vi "Nested Loops Solution.vi"() -> (3 "Solutions (Quantity)":i32[][](array[numeric]))   [LabVIEW 2014]
uses:
  ctl/Coin data--cluster.ctl
panel:
  in  "Update display?":bool
  out "No. solutions":i32
  out "Values (p)":i32[](array[numeric])
  out "Progress - current iteration values":i32[](array[numeric])
  out "Time taken (s)":dbl
  # "Beer money - Nested Loops/ Speedy solution"
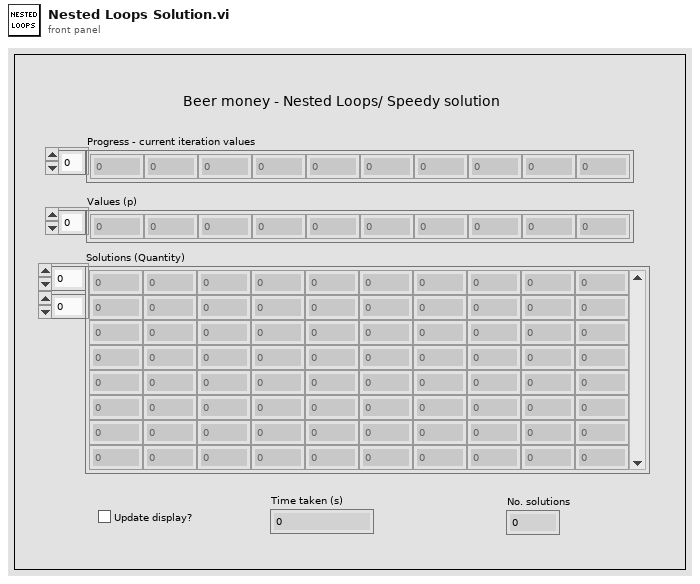
[diagram p1: front panel]
types:
  T1 = typedef "Coin data--cluster.ctl" = cluster{"Coin/note":i32, "Quantity":i32}
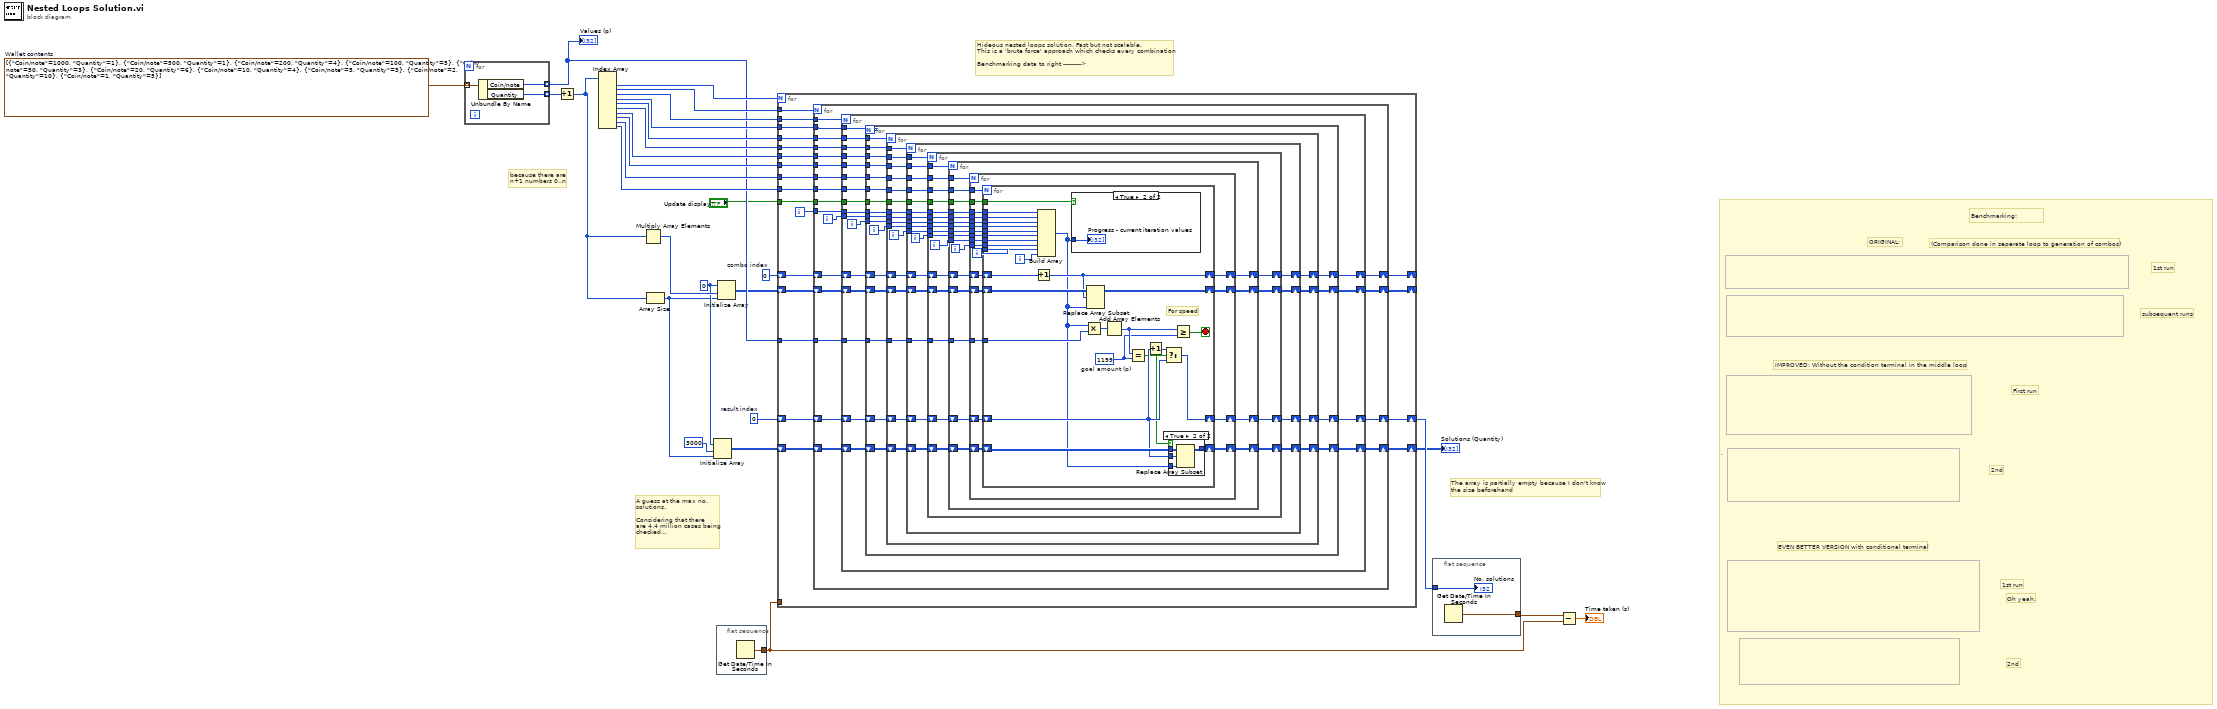
[diagram p0: block diagram]
diagram:
  w5 = 0 ("dimension size")
  w9 = 0  # result index
  w14 = 0  # combo index
  w28 = T1[] [{"Coin/note"=1000, "Quantity"=1}, {"Coin/note"=500, "Quantity"=1}, {"Coin/note"=200, "Quantity"=4}, {"Coin/note"=100, "Quantity"=5}, {"Coin/note"=50, "Quantity"=3}, {"Coin/note"=20, "Quantity"=6}, {"Coin/note"=10, "Quantity"=4}, {"Coin/note"=5, "Quantity"=3}, {"Coin/note"=2, "Quantity"=10}, {"Coin/note"=1, "Quantity"=5}]  # Wallet contents
  # "2nd"
  # "subsequent runs"
  # "The array is partially empty because I don't know\nthe size beforehand"
  # "Benchmarking:"
  # "(Comparison done in seperate loop to generation of combos)"
  # "1st run"
  # "Oh yeah."
  # "EVEN BETTER VERSION with conditional terminal"
  # "2nd"
  # "First run"
  # "IMPROVED: Without the condition terminal in the middle loop"
  # "A guess at the max no.\nsolutions.\n\nConsidering that there \nare 4.4 million cases being \nchecked..."
  # "ORIGINAL:"
  # "1st run"
  # "Hideous nested loops solution. Fast but not scalable.\nThis is a 'brute force' approach which checks every combination\n\nBenchmarking data to right --------->"
  # "because there are \nn+1 numbers 0..n"
  # "."
  n1 = for {
    tunnel: w28 -> [w31] mode=indexing
    tunnel: [w30] -> w10 mode=indexing
    tunnel: [w29] -> w27 mode=indexing
    n2 = Unbundle By Name(w31) -> ("Coin/note"=w30:i32, "Quantity"=w29:i32)
  }
  "Values (p)" <- w10
  n3 = Increment(x=w27) -> (x+1=w13:i32[])
  n4 = Index Array(array=w13) -> (element #1=w25:i32, element #2=w24:i32, element #3=w23:i32, element #4=w22:i32, element #5=w21:i32, element #6=w20:i32, element #7=w19:i32, element #8=w18:i32, element #9=w17:i32, element #10=w16:i32)  [unwired: 10 in]
  n5 = Multiply Array Elements(1:w13) -> (0:w26:i32)
  n6 = Array Size(array=w13) -> (size(s)=w4:i32)
  n7 = Initialize Array(w5, 3000 ("dimension size"), w4) -> (w6:i32[][])
  n8 = flat-sequence {
    tunnel: [w32] -> w15
    frame #0 {
      n9 = Get Date/Time In Seconds() -> (seconds since 1Jan1904=w32:timestamp)
    }
  }
  n10 = Initialize Array(w5, w26, w4) -> (w8:i32[][])
  n11 = for {
    N: w25 -> [_]
    tunnel: w24 -> [w48]
    tunnel: w23 -> [w49]
    tunnel: w22 -> [w50]
    tunnel: w21 -> [w47]
    tunnel: w20 -> [w46]
    tunnel: w19 -> [w45]
    tunnel: w18 -> [w44]
    tunnel: w17 -> [w43]
    tunnel: w16 -> [w42]
    shift-right: [w52] -> _
    shift-left: w8 -> [w41]
    tunnel: w15 -> [_]
    shift-right: [w39] -> _
    shift-left: w14 -> [w40]
    tunnel: w10 -> [w38]
    shift-right: [w34] -> w7
    shift-left: w9 -> [w37]
    shift-right: [w35] -> w2
    shift-left: w6 -> [w36]
    tunnel: "Update display?" -> [w33]
    i -> [w51]
    n12 = for {
      N: w48 -> [_]
      tunnel: w51 -> [w72]
      tunnel: w49 -> [w68]
      tunnel: w50 -> [w69]
      tunnel: w47 -> [w67]
      tunnel: w46 -> [w66]
      tunnel: w45 -> [w65]
      tunnel: w44 -> [w64]
      tunnel: w43 -> [w63]
      tunnel: w42 -> [w62]
      shift-right: [w71] -> w52
      shift-left: w41 -> [w61]
      shift-right: [w59] -> w39
      shift-left: w40 -> [w60]
      tunnel: w38 -> [w58]
      shift-right: [w54] -> w34
      shift-left: w37 -> [w57]
      shift-right: [w55] -> w35
      shift-left: w36 -> [w56]
      tunnel: w33 -> [w53]
      i -> [w70]
      n13 = for {
        N: w68 -> [_]
        tunnel: w72 -> [w92]
        tunnel: w70 -> [w91]
        tunnel: w69 -> [w88]
        tunnel: w67 -> [w87]
        tunnel: w66 -> [w86]
        tunnel: w65 -> [w85]
        tunnel: w64 -> [w84]
        tunnel: w63 -> [w83]
        tunnel: w62 -> [w82]
        shift-right: [w90] -> w71
        shift-left: w61 -> [w81]
        shift-right: [w79] -> w59
        shift-left: w60 -> [w80]
        tunnel: w58 -> [w78]
        shift-right: [w74] -> w54
        shift-left: w57 -> [w77]
        shift-right: [w75] -> w55
        shift-left: w56 -> [w76]
        tunnel: w53 -> [w73]
        i -> [w89]
        n14 = for {
          N: w88 -> [_]
          tunnel: w92 -> [w112]
          tunnel: w89 -> [w111]
          tunnel: w91 -> [w110]
          shift-right: [w109] -> w90
          shift-left: w81 -> [w108]
          tunnel: w87 -> [w107]
          tunnel: w86 -> [w106]
          tunnel: w85 -> [w105]
          tunnel: w84 -> [w104]
          tunnel: w83 -> [w103]
          tunnel: w82 -> [w102]
          shift-right: [w99] -> w79
          shift-left: w80 -> [w100]
          tunnel: w78 -> [w98]
          shift-right: [w94] -> w74
          shift-left: w77 -> [w97]
          shift-right: [w95] -> w75
          shift-left: w76 -> [w96]
          tunnel: w73 -> [w93]
          i -> [w101]
          n15 = for {
            N: w107 -> [_]
            tunnel: w112 -> [w132]
            tunnel: w111 -> [w131]
            tunnel: w110 -> [w130]
            shift-right: [w129] -> w109
            shift-left: w108 -> [w128]
            tunnel: w106 -> [w127]
            tunnel: w105 -> [w126]
            tunnel: w104 -> [w125]
            tunnel: w103 -> [w124]
            tunnel: w102 -> [w123]
            tunnel: w101 -> [w121]
            shift-right: [w119] -> w99
            shift-left: w100 -> [w120]
            tunnel: w98 -> [w118]
            shift-right: [w114] -> w94
            shift-left: w97 -> [w117]
            shift-right: [w115] -> w95
            shift-left: w96 -> [w116]
            tunnel: w93 -> [w113]
            i -> [w122]
            n16 = for {
              N: w127 -> [_]
              tunnel: w132 -> [w152]
              tunnel: w131 -> [w151]
              tunnel: w130 -> [w150]
              shift-right: [w149] -> w129
              shift-left: w128 -> [w148]
              tunnel: w126 -> [w147]
              tunnel: w125 -> [w146]
              tunnel: w124 -> [w145]
              tunnel: w123 -> [w144]
              tunnel: w122 -> [w143]
              tunnel: w121 -> [w141]
              shift-right: [w139] -> w119
              shift-left: w120 -> [w140]
              tunnel: w118 -> [w138]
              shift-right: [w134] -> w114
              shift-left: w117 -> [w137]
              shift-right: [w135] -> w115
              shift-left: w116 -> [w136]
              tunnel: w113 -> [w133]
              i -> [w142]
              n17 = for {
                N: w147 -> [_]
                tunnel: w152 -> [w172]
                tunnel: w151 -> [w171]
                tunnel: w150 -> [w170]
                shift-right: [w169] -> w149
                shift-left: w148 -> [w168]
                tunnel: w146 -> [w167]
                tunnel: w145 -> [w166]
                tunnel: w144 -> [w165]
                tunnel: w143 -> [w164]
                tunnel: w142 -> [w163]
                tunnel: w141 -> [w161]
                shift-right: [w159] -> w139
                shift-left: w140 -> [w160]
                tunnel: w138 -> [w158]
                shift-right: [w154] -> w134
                shift-left: w137 -> [w157]
                shift-right: [w155] -> w135
                shift-left: w136 -> [w156]
                tunnel: w133 -> [w153]
                i -> [w162]
                n18 = for {
                  N: w167 -> [_]
                  tunnel: w172 -> [w192]
                  tunnel: w171 -> [w191]
                  tunnel: w170 -> [w190]
                  shift-right: [w189] -> w169
                  shift-left: w168 -> [w188]
                  tunnel: w166 -> [w187]
                  tunnel: w165 -> [w186]
                  tunnel: w164 -> [w185]
                  tunnel: w163 -> [w184]
                  tunnel: w162 -> [w183]
                  tunnel: w161 -> [w181]
                  shift-right: [w179] -> w159
                  shift-left: w160 -> [w180]
                  tunnel: w158 -> [w178]
                  shift-right: [w174] -> w154
                  shift-left: w157 -> [w177]
                  shift-right: [w175] -> w155
                  shift-left: w156 -> [w176]
                  tunnel: w153 -> [w173]
                  i -> [w182]
                  n19 = for {
                    N: w187 -> [_]
                    tunnel: w192 -> [w212]
                    tunnel: w191 -> [w211]
                    tunnel: w190 -> [w210]
                    shift-right: [w209] -> w189
                    shift-left: w188 -> [w208]
                    tunnel: w186 -> [w207]
                    tunnel: w185 -> [w206]
                    tunnel: w184 -> [w205]
                    tunnel: w183 -> [w204]
                    tunnel: w182 -> [w203]
                    tunnel: w181 -> [w201]
                    shift-right: [w199] -> w179
                    shift-left: w180 -> [w200]
                    tunnel: w178 -> [w198]
                    shift-right: [w194] -> w174
                    shift-left: w177 -> [w197]
                    shift-right: [w195] -> w175
                    shift-left: w176 -> [w196]
                    tunnel: w173 -> [w193]
                    i -> [w202]
                    n20 = for {
                      N: w207 -> [_]
                      tunnel: w212 -> [w239]
                      tunnel: w211 -> [w238]
                      tunnel: w210 -> [w237]
                      shift-right: [w228] -> w209
                      shift-left: w208 -> [w229]
                      tunnel: w206 -> [w231]
                      tunnel: w205 -> [w230]
                      tunnel: w204 -> [w236]
                      tunnel: w203 -> [w235]
                      tunnel: w202 -> [w234]
                      tunnel: w201 -> [w232]
                      shift-right: [w226] -> w199
                      shift-left: w200 -> [w227]
                      tunnel: w198 -> [w224]
                      shift-right: [w222] -> w194
                      shift-left: w197 -> [w219]
                      shift-right: [w221] -> w195
                      shift-left: w196 -> [w220]
                      tunnel: w193 -> [w214]
                      i -> [w233]
                      stop <- w213 stop-if-true
                      w217 = 1199  # goal amount (p)
                      # "For speed"
                      n21 = Increment(x=w227) -> (x+1=w226:i32)
                      n22 = Build Array(w239, w237, w238, w232, w231, w230, w236, w235, w234, w233) -> (w216:i32[])
                      n23 = case shown="True" w214 {
                        tunnel: w216 -> [_ w240]
                        frame False {
                          # "Don't update display"
                        }
                        frame True {
                          "Progress - current iteration values" <- w240
                        }
                      }
                      n24 = Multiply(x=w216, y=w224) -> (x*y=w225:i32[])
                      n25 = Replace Array Subset(array=w229, new element=w216, index (row)=w226) -> (w228:i32[][])  [unwired: 1 in]
                      n26 = Add Array Elements(numeric array=w225) -> (sum=w218:i32)
                      n27 = Equal?(x=w218, y=w217) -> (x = y?=w215:bool)
                      n28 = Increment(x=w219) -> (x+1=w223:i32)
                      n29 = Select(t=w223, s=w215, f=w219) -> (s? t:f=w222:i32)
                      n30 = case shown="True" w215 {
                        tunnel: [w241 w245] -> w221
                        tunnel: w220 -> [w241 w244]
                        tunnel: w216 -> [_ w243]
                        tunnel: w219 -> [_ w242]
                        frame False {
                        }
                        frame True {
                          n31 = Replace Array Subset(array=w244, new element=w243, index (row)=w242) -> (w245:i32[][])  [unwired: 1 in]
                        }
                      }
                      n32 = Greater Or Equal?(x=w218, y=w217) -> (x >= y?=w213:bool)
                    }
                  }
                }
              }
            }
          }
        }
      }
    }
  }
  "Solutions (Quantity)" <- w2
  n33 = flat-sequence {
    tunnel: [w247] -> w12
    tunnel: w7 -> [w246]
    frame #0 {
      n34 = Get Date/Time In Seconds() -> (seconds since 1Jan1904=w247:timestamp)
      "No. solutions" <- w246
    }
  }
  n35 = Subtract(x=w12, y=w15) -> (x-y=→"Time taken (s)":dbl)
